vi "CameraStream.vi"() -> ()   [LabVIEW 2019]
uses:
  <vilib>/userdefined/High Color/IMAQdx.ctl
  <vilib>/vision/driver/NI_Vision_Acquisition_Software.lvlib
panel:
  in  "Session In":T1
  out "Image":T2(plugin-control)
  in  "Stop":bool
  # "e"
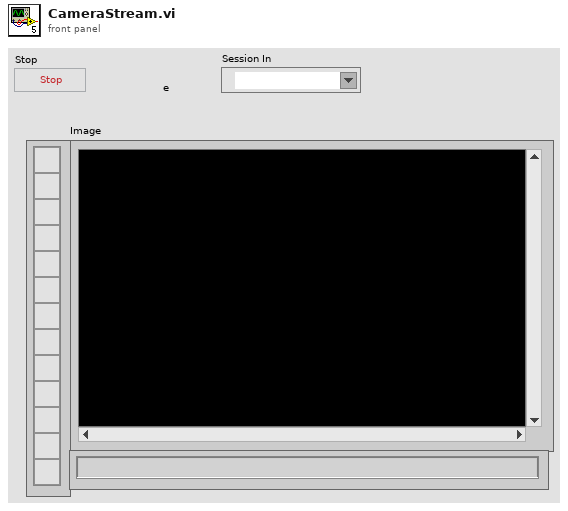
[diagram p1: front panel]
types:
  T1 = typedef "IMAQdx.ctl" = refnum<k21>
  T2 = typedef "IMAQ Image.ctl" = refnum<image>
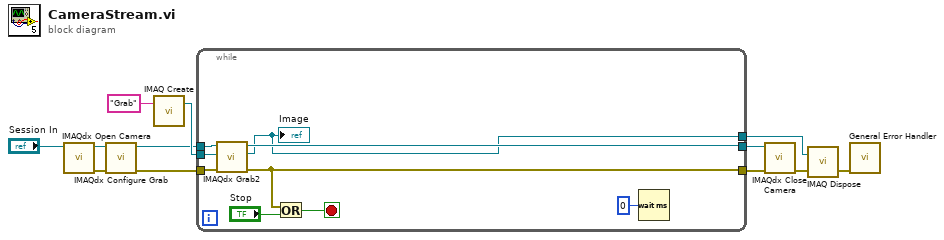
[diagram p0: block diagram]
diagram:
  n1 = call <vilib>:"IMAQdx Open Camera.vi"("Session In"="Session In") -> ("error out"=w10:errorcluster, "Session Out"=w12:T1)  [unwired: 9 in]
  n2 = call <vilib>:"IMAQdx Configure Grab.vi"("error in"=w10, "Session In"=w12) -> ("error out"=w1:errorcluster, "Session Out"=w2:T1)  [unwired: 8 in]
  n3 = call "IMAQ Create"("Image Name"="Grab") -> ("New Image"=w9:T2)  [unwired: 4 in, 1 out]
  n4 = while {
    tunnel: w1 -> [w14]
    tunnel: w9 -> [w18]
    tunnel: w2 -> [w17]
    tunnel: [w13] -> w7
    tunnel: [w15] -> w8
    tunnel: [w16] -> w6
    stop <- w20 stop-if-true
    n5 = call <vilib>:"IMAQdx Grab2.vi"("error in"=w14, "Image In"=w18, "Session In"=w17) -> ("error out"=w13:errorcluster, "Image Out"=w15:T2, "Session Out"=w16:T1)  [unwired: 5 in, 1 out]
    "Image" <- w15
    n6 = Or(x=w13, y="Stop") -> (x .or. y?=w20:bool)
    n7 = Wait (ms)(milliseconds to wait=u32 0) -> ()  [unwired: 1 out]
  }
  n8 = call <vilib>:"IMAQdx Close Camera.vi"("error in"=w7, "Session In"=w6) -> ("error out"=w5:errorcluster)  [unwired: 9 in]
  n9 = call "IMAQ Dispose"("Image"=w8, "error in (no error)"=w5) -> ("error out"=w4:errorcluster)  [unwired: 4 in]
  n10 = call <vilib>:"General Error Handler.vi"("error in (no error)"=w4) -> ()  [unwired: 10 in, 5 out]
